vi "Photon Counter Take Data - barebones2.vi"() -> ()   [LabVIEW 2009]
uses:
  SR400/SR400.lvlib
panel:
  out "ChB":dbl
  out "ChA":dbl
  in  "error in (no error)":errorcluster
  out "error out":errorcluster
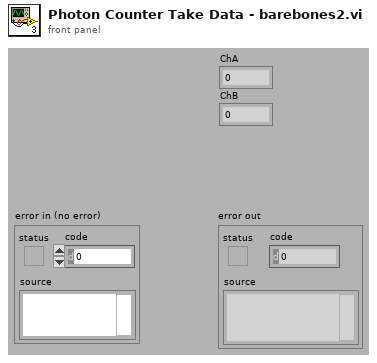
[diagram p1: front panel]
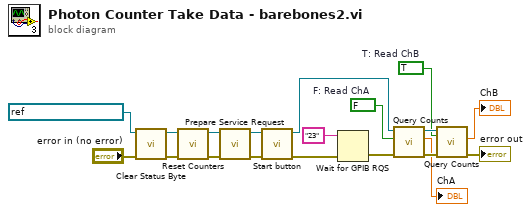
[diagram p0: block diagram]
diagram:
  w10 = TRUE  # T: Read ChB
  w11 = FALSE  # F: Read ChA
  n1 = call "Clear Status Byte.vi"("error in (no error)"="error in (no error)", "VISA resource name"=refnum<visa-resource-name> "GPIB0::23::INSTR") -> ("error out"=w14:errorcluster, "VISA resource name out"=w17:refnum<visa-resource-name>)  [unwired: 8 out]
  n2 = call "Reset Counters.vi"("error in (no error)"=w14, "VISA resource name"=w17) -> ("error out"=w13:errorcluster, "VISA resource name out"=w16:refnum<visa-resource-name>)  [unwired: 8 out]
  n3 = call "Prepare Service Request.vi"("error in (no error)"=w13, "VISA resource name"=w16) -> ("error out"=w12:errorcluster, "VISA resource name out"=w15:refnum<visa-resource-name>)  [unwired: 1 in, 7 out]
  n4 = call "Start button.vi"("error in (no error)"=w12, "VISA resource name"=w15) -> ("error out"=w4:errorcluster, "VISA resource name out"=w3:refnum<visa-resource-name>)  [unwired: 8 out]
  n5 = Wait for GPIB RQS(2:w4, 4:"23" ("address string")) -> (0:w2:errorcluster)  [unwired: 2 out]
  n6 = call "Query Counts.vi"("error in (no error)"=w2, "Read B?"=w11, "VISA resource name"=w3) -> ("error out"=w18:errorcluster, "Counts"=→"ChA":dbl, "VISA resource name out"=w19:refnum<visa-resource-name>)  [unwired: 6 out]
  n7 = call "Query Counts.vi"("error in (no error)"=w18, "Read B?"=w10, "VISA resource name"=w19) -> ("error out"=→"error out":errorcluster, "Counts"=→"ChB":dbl)  [unwired: 7 out]
